vi "New Array Child.vi"(7 "Value Type (String)":T1, 8 "error in (no error)":errorcluster, 10 "Array Parent":refnum<class "Config Element.lvclass">, 11 "Config Manager in":refnum<class "Config Manager.lvclass">) -> (0 "error out":errorcluster, 1 "New Child":refnum<class "Config Element.lvclass">, 2 "Child Index":i32, 3 "Config Manager out":refnum<class "Config Manager.lvclass">)   [LabVIEW 2023, in "CDM-Config.lvlib" / "Config Manager.lvclass"]
doc: "Creates a new element directly under the specified parent element with the specified name. All direct children of an element must have unique names. Additionally, children cannot be named \"Meta\" as that is reserved for persisting and loading configs."
uses:
  Config Manager.lvclass
  Config Element/Config Element.lvclass
  Value Type.ctl
  Config Manager.lvclass/Config Manager.ctl
  CDM-Config.lvlib
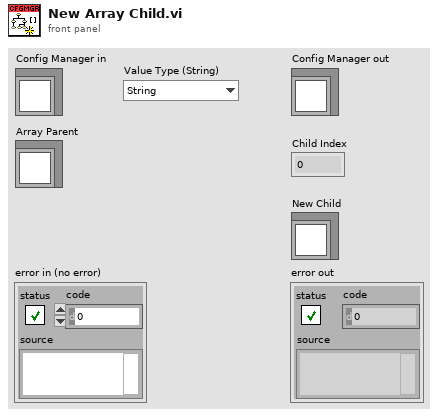
[diagram p1: front panel]
types:
  T1 = typedef "CDM-Config.lvlib/Value Type.ctl" = enum16{"String", "Number", "Bool", "Object", "Array"}
  T2 = typedef "CDM-Config.lvlib/Config Manager.lvclass/Ref Data.ctl" = cluster{"Elements":refnum<class "Config Element.lvclass">[], "Hierarchy Map":map{string[], i32}, "Element Map":map{refnum<class "Config Element.lvclass">, i32}}
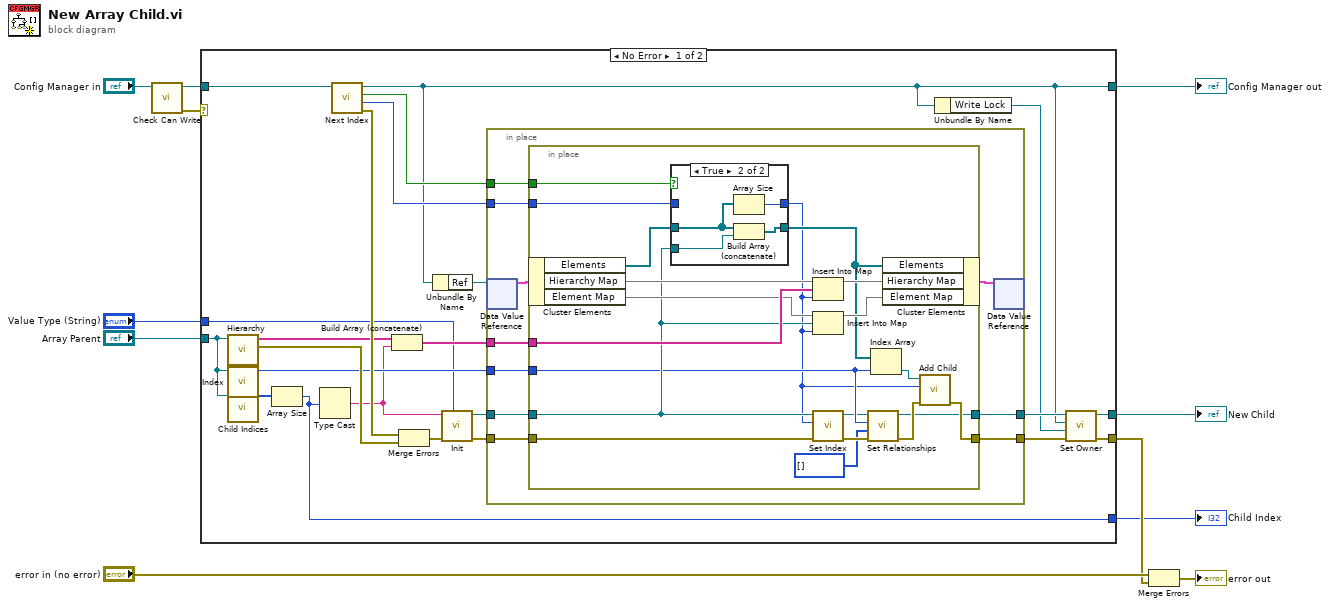
[diagram p0: block diagram]
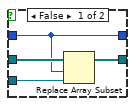
[diagram p2: hidden frame]
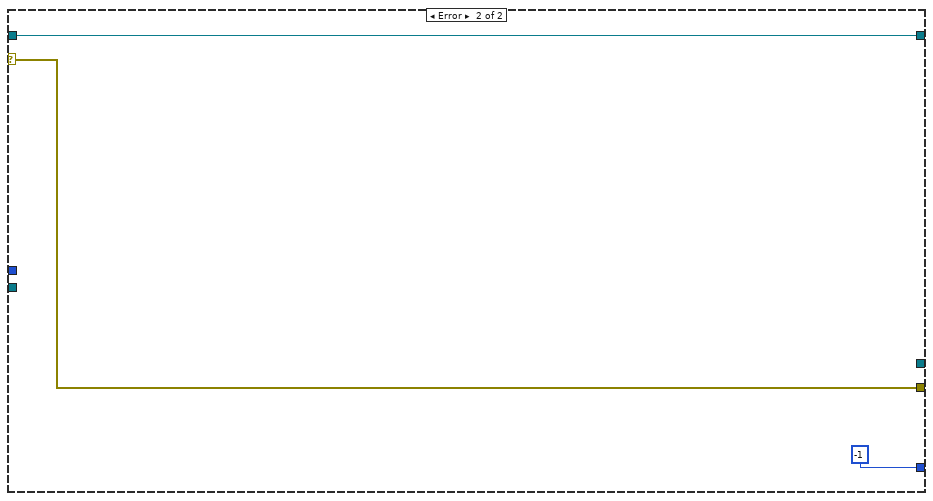
[diagram p3: hidden frame]
diagram:
  n1 = call "Check Can Write.vi"("Config Manager in"="Config Manager in") -> ("error out"=w1:errorcluster, "Config Manager out"=w2:refnum<class "Config Manager.lvclass">)  [unwired: 9 in]
  n2 = case shown="No Error" w1 {
    selector: w1 -> [_ w74]
    tunnel: w2 -> [w34 w73]
    tunnel: [w33 _] -> w9
    tunnel: [w13 w73] -> w8
    tunnel: [w32 w74] -> w6
    tunnel: "Array Parent" -> [w18 _]
    tunnel: [w16 -1] -> w4
    tunnel: "Value Type (String)" -> [w14 _]
    frame No Error {
      n3 = call "Hierarchy.vi"("Config Element in"=w18) -> ("error out"=w30:errorcluster, "Hierarchy"=w29:string[])  [unwired: 9 in]
      n4 = call "Index.vi"("Config Element in"=w18) -> ("Index"=w25:i32)  [unwired: 9 in, 1 out]
      n5 = call "Child Indices.vi"("Config Element in"=w18) -> ("Children"=w17:i32[])  [unwired: 9 in, 1 out]
      n6 = Array Size(array=w17) -> (size(s)=w16:i32)
      n7 = Type Cast(x=w16) -> (*(type *) &x=w15:string)  [unwired: 1 in]
      n8 = call "Next Index.vi"("Config Manager in"=w34) -> ("error out"=w31:errorcluster, "Index"=w24:i32, "Add to End"=w23:bool, "Config Manager out"=w13:refnum<class "Config Manager.lvclass">)  [unwired: 7 in]
      n9 = Build Array (concatenate)(w29, w15) -> (w26:string[])
      n10 = Merge Errors(w31, w30) -> (w21:errorcluster)
      n11 = Unbundle By Name(w13) -> ("Ref"=w28:refnum<data-value>)
      n12 = call "Init.vi"("Value Type"=w14, "error in (no error)"=w21, "Name"=w15) -> ("error out"=w20:errorcluster, "Config Element out"=w27:refnum<class "Config Element.lvclass">)  [unwired: 7 in]
      n13 = in-place {
        in-place-border: w27 -> [w42]
        in-place-border: w26 -> [w41]
        in-place-border: [w40] -> w22
        in-place-border: w25 -> [w39]
        in-place-border: w24 -> [w38]
        in-place-border: w23 -> [w37]
        in-place-border: w20 -> [w36]
        in-place-border: [w35] -> w19
        n14 = in-place-dvr #1(w28) -> (w44:T2)  [unwired: 1 out]
        n15 = in-place {
          in-place-border: w42 -> [w55]
          in-place-border: w41 -> [w59]
          in-place-border: [w50] -> w40
          in-place-border: w39 -> [w49]
          in-place-border: w38 -> [w52]
          in-place-border: w37 -> [w51]
          in-place-border: w36 -> [w45]
          in-place-border: [w63] -> w35
          n16 = in-place-cluster #2(w44) -> ("Elements"=w61:refnum<class "Config Element.lvclass">[], "Hierarchy Map"=w60:map{string[], i32}, "Element Map"=w58:map{refnum<class "Config Element.lvclass">, i32})
          n17 = case shown="True" w51 {
            tunnel: w61 -> [w68 w69]
            tunnel: w55 -> [w67 w72]
            tunnel: [w66 w71] -> w54
            tunnel: [w65 w70] -> w46
            tunnel: w52 -> [w65 _]
            frame False {
              n18 = Replace Array Subset(array=w68, new element=w67, index=w65) -> (w66:refnum<class "Config Element.lvclass">[])
            }
            frame True {
              n19 = Array Size(array=w69) -> (size(s)=w70:i32)
              n20 = Build Array (concatenate)(w69, w72) -> (w71:refnum<class "Config Element.lvclass">[])
            }
          }
          n21 = Insert Into Map(map in=w60, key=w59, value=w46) -> (map out=w57:map{string[], i32})  [unwired: 2 out]
          n22 = Insert Into Map(map in=w58, key=w55, value=w46) -> (map out=w56:map{refnum<class "Config Element.lvclass">, i32})  [unwired: 2 out]
          n23 = call "Set Index.vi"("error in (no error)"=w45, "Index"=w46, "Config Element in"=w55) -> ("error out"=w62:errorcluster, "Config Element out"=w47:refnum<class "Config Element.lvclass">)  [unwired: 7 in]
          n24 = call "Set Relationships.vi"("error in (no error)"=w62, "Children"=i32[] [], "Parent"=w49, "Config Element in"=w47) -> ("error out"=w64:errorcluster, "Config Element out"=w50:refnum<class "Config Element.lvclass">)  [unwired: 6 in]
          n25 = Index Array(array=w54, index=w49) -> (element=w53:refnum<class "Config Element.lvclass">)
          n26 = in-place-cluster #2("Elements"=w54, "Hierarchy Map"=w57, "Element Map"=w56) -> (w43:T2)
          n27 = call "Add Child.vi"("error in (no error)"=w64, "Child"=w46, "Config Element in"=w53) -> ("error out"=w63:errorcluster)  [unwired: 7 in, 1 out]
        }
        n28 = in-place-dvr #1(w43) -> ()  [unwired: 2 out]
      }
      n29 = Unbundle By Name(w13) -> ("Write Lock"=w12:refnum<notifier>)
      n30 = call "Set Owner.vi"("error in (no error)"=w19, "Write Lock"=w12, "Owner"=w13, "Config Element in"=w22) -> ("error out"=w32:errorcluster, "Config Element out"=w33:refnum<class "Config Element.lvclass">)  [unwired: 6 in]
    }
    frame Error {
    }
  }
  "Config Manager out" <- w8
  "New Child" <- w9
  "Child Index" <- w4
  n31 = Merge Errors("error in (no error)", w6) -> (→"error out":errorcluster)
